vi "convert hex to string.vi"(1 "hex":u32 format="%.0x") -> (0 "string":string)   [LabVIEW 2021, in "TSC Material Theme.lvlib"]
doc: "convert a hex value to an ARGB text string\n\n<b>Code Developed By:</b>\nTechnology Service Corporation\nwww.tsc.com/atcs\n\nDeveloper:\nDaniel Coons"
uses:
  TSC Material Theme.lvlib
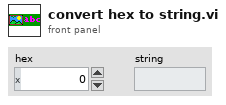
[diagram p1: front panel]
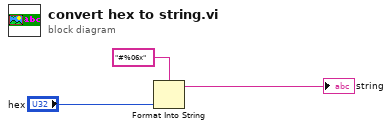
[diagram p0: block diagram]
diagram:
  n1 = Format Into String(format string="#%06x", "hex") -> (resulting string=→"string":string)  [unwired: 2 in, 1 out]
